vi "Post-Bury Hook.vi"(8 "Error In":errorcluster) -> (0 "Error Out":errorcluster)   [LabVIEW 2018, in "Tests.lvlib" / "Toolkit.lvlib" / "Integration.lvlib"]
uses:
  Integration.lvlib
  Support/Bury Target.vi
  Hooks/Post-Bury.vi
  src/Toolkit/Toolkit.lvlib
  <vilib>/addons/_JKI Toolkits/Caraya/classes/Test/Test.lvclass
  Tests.lvlib
  <vilib>/addons/_JKI Toolkits/Caraya/classes/Assert/Assert.lvclass
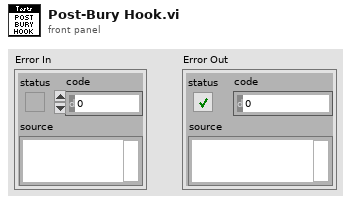
[diagram p1: front panel]
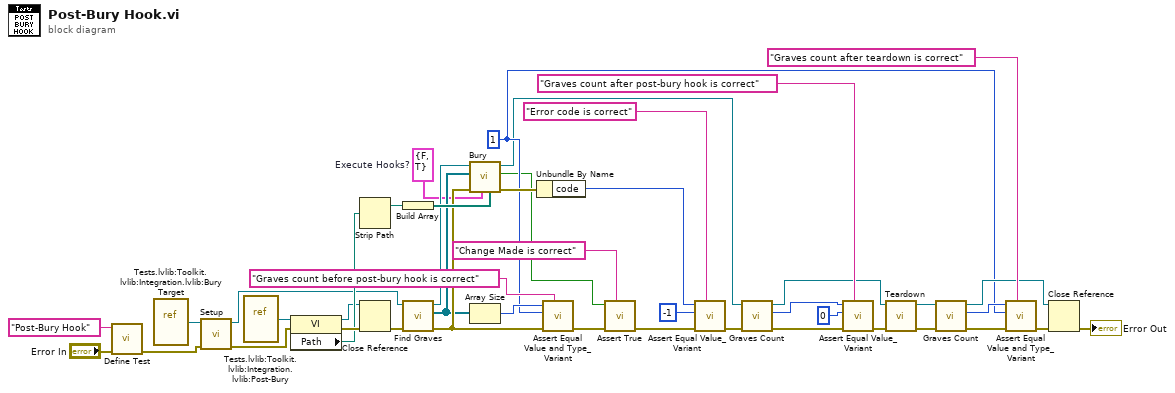
[diagram p0: block diagram]
diagram:
  w6 = cluster{"Pre":bool, "Post":bool} {"Pre"=FALSE, "Post"=TRUE}  # Execute Hooks?
  w10 = 1 ("size(s)")
  n1 = call <vilib>:"Define Test.vi"("error in (no error)"="Error In", "Label (VI Title)"="Post-Bury Hook") -> ("error out"=w39:errorcluster)  [unwired: 9 in]
  n2 = vi-ref "Tests.lvlib:Toolkit.lvlib:Integration.lvlib:Bury Target.vi"() -> (w21:refnum<vi>)
  n3 = call "Setup.vi"("Error In"=w39, "VI In"=w21) -> ("Error Out"=w29:errorcluster, "VI Out"=w19:refnum<vi>)  [unwired: 8 in]
  n4 = vi-ref "Tests.lvlib:Toolkit.lvlib:Integration.lvlib:Post-Bury.vi"() -> (w1:refnum<vi>)
  n5 = property class="VI"(reference=w1, error in=w29) -> (reference out=w25:refnum<vi>, error out=w28:errorcluster, "Path"=w27:path)
  n6 = Strip Path(path=w27) -> (stripped path=w26:path)  [unwired: 1 out]
  n7 = Close Reference(reference=w25, error in (no error)=w28) -> (error out=w20:errorcluster)
  n8 = Build Array(w26) -> (w22:path[])
  n9 = call "Find Graves.vi"("Error In"=w20, "VI In"=w19) -> ("Error Out"=w17:errorcluster, "Graves"=w16:refnum<vi>[], "VI Out"=w18:refnum<vi>)  [unwired: 7 in]
  n10 = call "Bury.vi"("Hook Search Path"=w22, "Execute Hooks?"=w6, "Error In"=w17, "Graves"=w16, "VI In"=w18) -> ("Error Out"=w14:errorcluster, "Change Made?"=w3:bool, "VI Out"=w8:refnum<vi>)  [unwired: 4 in]
  n11 = Array Size(array=w16) -> (size(s)=w15:i32)
  n12 = Unbundle By Name(w14) -> ("code"=w24:i32)
  n13 = call <vilib>:"Assert Equal Value and Type_Variant.vi"("Label"="Graves count before post-bury hook is correct", "error in (no error)"=w17, "Y"=w10, "X"=w15) -> ("error out"=w38:errorcluster)  [unwired: 7 in]
  n14 = call <vilib>:"Assert True.vi"("Label"="Change Made is correct", "error in (no error)"=w38, "True?"=w3) -> ("error out"=w4:errorcluster)  [unwired: 8 in]
  n15 = call <vilib>:"Assert Equal Value_Variant.vi"("Label"="Error code is correct", "error in (no error)"=w4, "Y"=-1 ("code"), "X"=w24) -> ("error out"=w13:errorcluster)  [unwired: 7 in]
  n16 = call "Graves Count.vi"("Error In"=w13, "Test Target In"=w8) -> ("Error Out"=w12:errorcluster, "Graves Count"=w11:i32, "Test Target Out"=w9:refnum<vi>)  [unwired: 7 in]
  n17 = call <vilib>:"Assert Equal Value_Variant.vi"("Label"="Graves count after post-bury hook is correct", "error in (no error)"=w12, "Y"=0 ("Graves Count"), "X"=w11) -> ("error out"=w7:errorcluster)  [unwired: 7 in]
  n18 = call "Teardown.vi"("Error In"=w7, "VI In"=w9) -> ("Error Out"=w32:errorcluster, "VI Out"=w34:refnum<vi>)  [unwired: 8 in]
  n19 = call "Graves Count.vi"("Error In"=w32, "Test Target In"=w34) -> ("Error Out"=w31:errorcluster, "Graves Count"=w30:i32, "Test Target Out"=w33:refnum<vi>)  [unwired: 7 in]
  n20 = call <vilib>:"Assert Equal Value and Type_Variant.vi"("Label"="Graves count after teardown is correct", "error in (no error)"=w31, "Y"=w10, "X"=w30) -> ("error out"=w36:errorcluster)  [unwired: 7 in]
  n21 = Close Reference(reference=w33, error in (no error)=w36) -> (error out=→"Error Out":errorcluster)
